vi "Read Waveform (Min Max).vi"(8 "error in (no error)":errorcluster, 9 "Maximum Time (10000 ms)":u32=10000, 10 "Channel (1: Channel 1)":u16(ring)=1 items=["Channel 1"=1, "Channel 2"=2, "Channel 3"=3, "Channel 4"=4], 11 "VISA resource name":refnum<visa-resource-name>) -> (0 "error out":errorcluster, 1 "Max Waveform Data":waveform(dbl)(graph), 2 "Min Waveform Data":waveform(dbl)(graph), 3 "VISA resource name out":refnum<visa-resource-name>)   [LabVIEW 2011, in "Agilent DSO1000 Series.lvlib"]
doc: "Initiates an acquisition on the channels that you enable with the Configure Channel.vi. It then waits for the acquisition to complete, and returns the min/max waveforms for the channel you specify. You call the Fetch Min Max Waveform.vi to obtain the min/max waveforms for each of the remaining enabled channels without initiating another acquisition.\n\nUse this VI to read waveforms when you set the acquisition type to \"Peak Detect\".\n\n<B>Notes:</B>\n\n(1) After this VI executes, each element in the Min Waveform Array and Max Waveform Array parameters is either a voltage or a value indicating that the oscilloscope could not sample a voltage."
uses:
  <instrlib>/Agilent DSO1000 Series/Agilent DSO1000 Series.lvlib
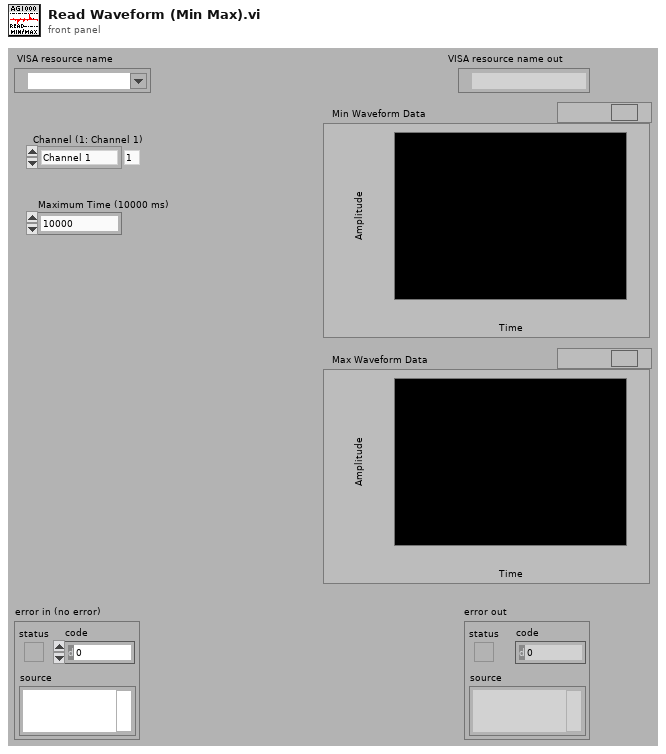
[diagram p1: front panel]
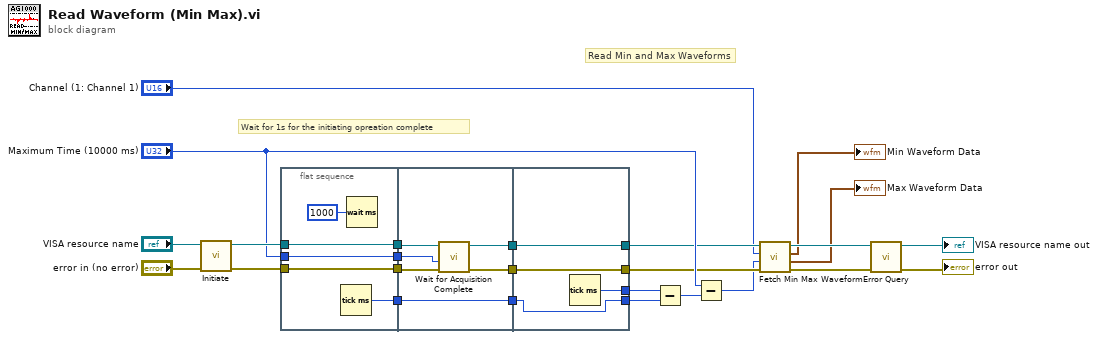
[diagram p0: block diagram]
diagram:
  # "Wait for 1s for the initiating opreation complete"
  # "Read Min and Max Waveforms"
  n1 = call <instrlib>:"Initiate.vi"("error in (no error)"="error in (no error)", "VISA resource name"="VISA resource name") -> ("error out"=w24:errorcluster, "VISA resource name out"=w25:refnum<visa-resource-name>)  [unwired: 8 in]
  n2 = flat-sequence {
    tunnel: w25 -> [w29]
    tunnel: [w29] -> w9
    tunnel: w24 -> [w28]
    tunnel: [w28] -> w8
    tunnel: [w30] -> w7
    tunnel: "Maximum Time (10000 ms)" -> [w27]
    tunnel: [w27] -> w6
    tunnel: w9 -> [w36]
    tunnel: [w35] -> w5
    tunnel: w8 -> [w34]
    tunnel: [w33] -> w4
    tunnel: w7 -> [w31]
    tunnel: [w31] -> w3
    tunnel: w6 -> [w32]
    tunnel: [w39] -> w17
    tunnel: w5 -> [w39]
    tunnel: [w38] -> w14
    tunnel: w4 -> [w38]
    tunnel: [w37] -> w22
    tunnel: w3 -> [w37]
    tunnel: [w40] -> w21
    frame #0 {
      n3 = Tick Count (ms)() -> (millisecond timer value=w30:u32)
      n4 = Wait (ms)(milliseconds to wait=u32 1000) -> ()  [unwired: 1 out]
    }
    frame #1 {
      n5 = call <instrlib>:"Wait for Acquisition Complete.vi"("error in (no error)"=w34, "Maximum Time (10000 ms)"=w32, "VISA resource name"=w36) -> ("error out"=w33:errorcluster, "VISA resource name out"=w35:refnum<visa-resource-name>)  [unwired: 7 in]
    }
    frame #2 {
      n6 = Tick Count (ms)() -> (millisecond timer value=w40:u32)
    }
  }
  n7 = Subtract(x=w21, y=w22) -> (x-y=w23:u32)
  n8 = Subtract(x="Maximum Time (10000 ms)", y=w23) -> (x-y=w13:u32)
  n9 = call <instrlib>:"Fetch Min Max Waveform.vi"("error in (no error)"=w14, "Maximum Time (10000 ms)"=w13, "Channel (1: Channel 1)"="Channel (1: Channel 1)", "VISA resource name"=w17) -> ("error out"=w15:errorcluster, "Max Waveform Data"=→"Max Waveform Data":waveform(dbl), "Min Waveform Data"=→"Min Waveform Data":waveform(dbl), "VISA resource name out"=w16:refnum<visa-resource-name>)  [unwired: 4 in]
  n10 = call <instrlib>:"Error Query.vi"("error in (no error)"=w15, "VISA resource name"=w16) -> ("error out"=→"error out":errorcluster, "VISA resource name out"=→"VISA resource name out":refnum<visa-resource-name>)  [unwired: 6 in, 2 out]
